vi "RSA Decrypt.vi"(7 "private_key":string, 8 "error in (no error)":errorcluster, 10 "encrypted data":u8[](array[numeric]), 11 "RSA in":refnum<class "RSA.lvclass">) -> (0 "error out":errorcluster, 2 "data":u8[](array[numeric]), 3 "RSA out":refnum<class "RSA.lvclass">)   [LabVIEW 2023, in "RSA.lvclass"]
uses:
  RSA.lvclass
  RSA.lvclass/RSA.ctl
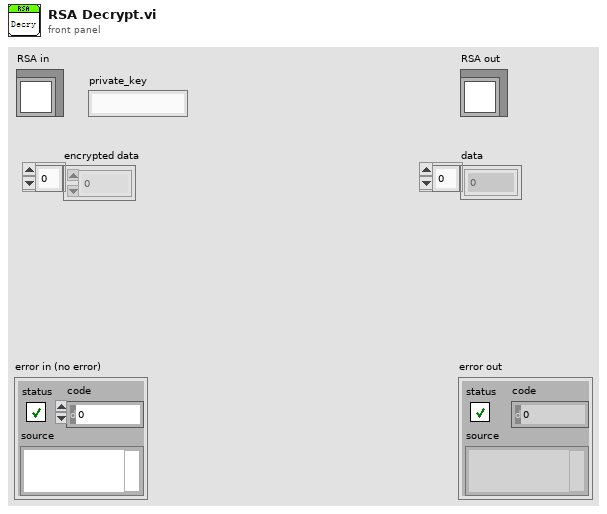
[diagram p1: front panel]
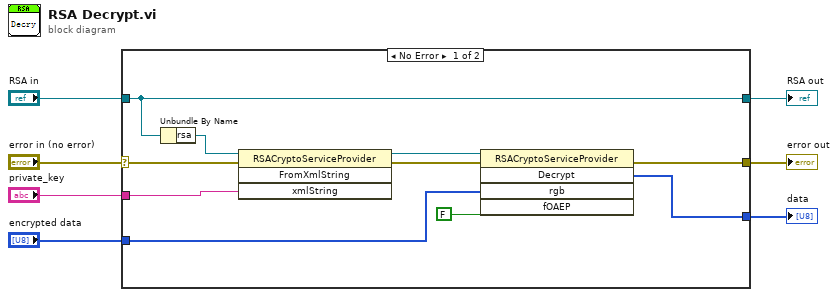
[diagram p0: block diagram]
diagram:
  n1 = case shown="No Error" "error in (no error)" {
    selector: "error in (no error)" -> [w11 w19]
    tunnel: [w9 w19] -> w6
    tunnel: [w13 w18] -> w4
    tunnel: "RSA in" -> [w13 w18]
    tunnel: "private_key" -> [w17 _]
    tunnel: "encrypted data" -> [w10 _]
    tunnel: [w8 _] -> w1
    frame No Error {
      n2 = Unbundle By Name(w13) -> ("rsa"=w12:refnum<k24>)
      n3 = invoke class="RSACryptoServiceProvider" method="FromXmlString"(reference=w12, error in=w11, "xmlString"=w17) -> (reference out=w15:refnum<k24>, error out=w16:errorcluster)  [unwired: 1 in, 2 out]
      n4 = invoke class="RSACryptoServiceProvider" method="Decrypt"(reference=w15, error in=w16, "rgb"=w10, "fOAEP"=FALSE) -> (error out=w9:errorcluster, "Decrypt"=w8:u8[])  [unwired: 1 in, 3 out]
    }
    frame Error {
    }
  }
  "error out" <- w6
  "RSA out" <- w4
  "data" <- w1
